vi "delete_curve.vi"(10 "簇":T23, 11 "配置":T1 {"串口通信UI"."Format" items=["标准帧", "扩展帧"]; "串口通信UI"."Type" items=["数据帧", "远程帧"]; "串口通信UI"."ID" format="0x%x"; "串口通信UI"."Fliter" items=["接收所有类型"=1, "只接收标准帧"=2, "只接收扩展帧"=3]; "串口通信UI"."kBaudRate" items=["5k bps"=1, "10k bps"=2, "20k bps"=3, "40k bps"=4, "50k bps"=5, "80k bps"=6, "100k bps"=7, "125k bps"=8, "200k bps"=9, "250k bps"=10, "400k bps"=11, "500k bps"=12, "666k bps"=13, "800k bps"=14, "1000k bps"=15, "33.33k bps"=16, "66.66k bps"=17, "83.33k bps"=18]; "串口通信UI"."Mode" items=["正常工作", "仅侦听模式", "自测模式（环回）"]; "串口通信UI"."InitFlag" items=["使用界面设置参数"=1]; "串口通信UI"."AccMask" format="%08x"; "串口通信UI"."AccCode" format="%08x"; "串口通信UI"."Channel" items=["通道1", "通道2"]; "串口通信UI"."DevType" items=["USB-CAN"=3, "USB-CAN2"=4]; "安全报警UI"."操作 8" items=["产生报警信息（不发声），等待手动操作", "产生报警信息（发声），等待手动操作", "产生报警信息（不发声），自动刹车", "产生报警信息（发声），自动刹车", "产生报警信息（不发声），立即自动断电，开启泄放电阻", "产生报警信息（发声），立即自动断电，开启泄放电阻"]; "安全报警UI"."操作 7" items=["产生报警信息（不发声），等待手动操作", "产生报警信息（发声），等待手动操作", "产生报警信息（不发声），自动刹车", "产生报警信息（发声），自动刹车", "产生报警信息（不发声），立即自动断电，开启泄放电阻", "产生报警信息（发声），立即自动断电，开启泄放电阻"]; "安全报警UI"."操作 6" items=["产生报警信息（不发声），等待手动操作", "产生报警信息（发声），等待手动操作", "产生报警信息（不发声），自动刹车", "产生报警信息（发声），自动刹车", "产生报警信息（不发声），立即自动断电，开启泄放电阻", "产生报警信息（发声），立即自动断电，开启泄放电阻"]; "安全报警UI"."操作 5" items=["产生报警信息（不发声），等待手动操作", "产生报警信息（发声），等待手动操作", "产生报警信息（不发声），自动刹车", "产生报警信息（发声），自动刹车", "产生报警信息（不发声），立即自动断电，开启泄放电阻", "产生报警信息（发声），立即自动断电，开启泄放电阻"]; "安全报警UI"."操作 4" items=["产生报警信息（不发声），等待手动操作", "产生报警信息（发声），等待手动操作", "产生报警信息（不发声），自动刹车", "产生报警信息（发声），自动刹车", "产生报警信息（不发声），立即自动断电，开启泄放电阻", "产生报警信息（发声），立即自动断电，开启泄放电阻"]; "安全报警UI"."操作 3" items=["产生报警信息（不发声），等待手动操作", "产生报警信息（发声），等待手动操作", "产生报警信息（不发声），自动刹车", "产生报警信息（发声），自动刹车", "产生报警信息（不发声），立即自动断电，开启泄放电阻", "产生报警信息（发声），立即自动断电，开启泄放电阻"]; "安全报警UI"."操作 2" items=["产生报警信息（不发声），等待手动操作", "产生报警信息（发声），等待手动操作", "产生报警信息（不发声），自动刹车", "产生报警信息（发声），自动刹车", "产生报警信息（不发声），立即自动断电，开启泄放电阻", "产生报警信息（发声），立即自动断电，开启泄放电阻"]; "安全报警UI"."操作" items=["产生报警信息（不发声），等待手动操作", "产生报警信息（发声），等待手动操作", "产生报警信息（不发声），自动刹车", "产生报警信息（发声），自动刹车", "产生报警信息（不发声），立即自动断电，开启泄放电阻", "产生报警信息（发声），立即自动断电，开启泄放电阻"]}) -> (3 "配置输出":T1 {"串口通信UI"."Format" items=["标准帧", "扩展帧"]; "串口通信UI"."Type" items=["数据帧", "远程帧"]; "串口通信UI"."ID" format="0x%x"; "串口通信UI"."Fliter" items=["接收所有类型"=1, "只接收标准帧"=2, "只接收扩展帧"=3]; "串口通信UI"."kBaudRate" items=["5k bps"=1, "10k bps"=2, "20k bps"=3, "40k bps"=4, "50k bps"=5, "80k bps"=6, "100k bps"=7, "125k bps"=8, "200k bps"=9, "250k bps"=10, "400k bps"=11, "500k bps"=12, "666k bps"=13, "800k bps"=14, "1000k bps"=15, "33.33k bps"=16, "66.66k bps"=17, "83.33k bps"=18]; "串口通信UI"."Mode" items=["正常工作", "仅侦听模式", "自测模式（环回）"]; "串口通信UI"."InitFlag" items=["使用界面设置参数"=1]; "串口通信UI"."AccMask" format="%08x"; "串口通信UI"."AccCode" format="%08x"; "串口通信UI"."Channel" items=["通道1", "通道2"]; "串口通信UI"."DevType" items=["USB-CAN"=3, "USB-CAN2"=4]; "安全报警UI"."操作 8" items=["产生报警信息（不发声），等待手动操作", "产生报警信息（发声），等待手动操作", "产生报警信息（不发声），自动刹车", "产生报警信息（发声），自动刹车", "产生报警信息（不发声），立即自动断电，开启泄放电阻", "产生报警信息（发声），立即自动断电，开启泄放电阻"]; "安全报警UI"."操作 7" items=["产生报警信息（不发声），等待手动操作", "产生报警信息（发声），等待手动操作", "产生报警信息（不发声），自动刹车", "产生报警信息（发声），自动刹车", "产生报警信息（不发声），立即自动断电，开启泄放电阻", "产生报警信息（发声），立即自动断电，开启泄放电阻"]; "安全报警UI"."操作 6" items=["产生报警信息（不发声），等待手动操作", "产生报警信息（发声），等待手动操作", "产生报警信息（不发声），自动刹车", "产生报警信息（发声），自动刹车", "产生报警信息（不发声），立即自动断电，开启泄放电阻", "产生报警信息（发声），立即自动断电，开启泄放电阻"]; "安全报警UI"."操作 5" items=["产生报警信息（不发声），等待手动操作", "产生报警信息（发声），等待手动操作", "产生报警信息（不发声），自动刹车", "产生报警信息（发声），自动刹车", "产生报警信息（不发声），立即自动断电，开启泄放电阻", "产生报警信息（发声），立即自动断电，开启泄放电阻"]; "安全报警UI"."操作 4" items=["产生报警信息（不发声），等待手动操作", "产生报警信息（发声），等待手动操作", "产生报警信息（不发声），自动刹车", "产生报警信息（发声），自动刹车", "产生报警信息（不发声），立即自动断电，开启泄放电阻", "产生报警信息（发声），立即自动断电，开启泄放电阻"]; "安全报警UI"."操作 3" items=["产生报警信息（不发声），等待手动操作", "产生报警信息（发声），等待手动操作", "产生报警信息（不发声），自动刹车", "产生报警信息（发声），自动刹车", "产生报警信息（不发声），立即自动断电，开启泄放电阻", "产生报警信息（发声），立即自动断电，开启泄放电阻"]; "安全报警UI"."操作 2" items=["产生报警信息（不发声），等待手动操作", "产生报警信息（发声），等待手动操作", "产生报警信息（不发声），自动刹车", "产生报警信息（发声），自动刹车", "产生报警信息（不发声），立即自动断电，开启泄放电阻", "产生报警信息（发声），立即自动断电，开启泄放电阻"]; "安全报警UI"."操作" items=["产生报警信息（不发声），等待手动操作", "产生报警信息（发声），等待手动操作", "产生报警信息（不发声），自动刹车", "产生报警信息（发声），自动刹车", "产生报警信息（不发声），立即自动断电，开启泄放电阻", "产生报警信息（发声），立即自动断电，开启泄放电阻"]})   [LabVIEW 2018, in "UI.lvlib"]
uses:
  UI.lvlib
  Settings/Settings.ctl
  Acquisition/Hardware Configuration.ctl
  Acquisition/Signal Type.ctl
  Logging/Logging Configuration.ctl
  Logging/Logging.lvlib
  Acquisition/Acquisition.lvlib
  Settings/Settings.lvlib
panel:
  # "参数配置文件"
  # "输入数据文件"
  # "加载电机"
  # "负载电机"
  # "注：每次运行实验时销毁现有所有图像"
  # "参数配置文件"
  # "输入数据文件"
  # "加载电机"
  # "负载电机"
  # "注：每次运行实验时销毁现有所有图像"
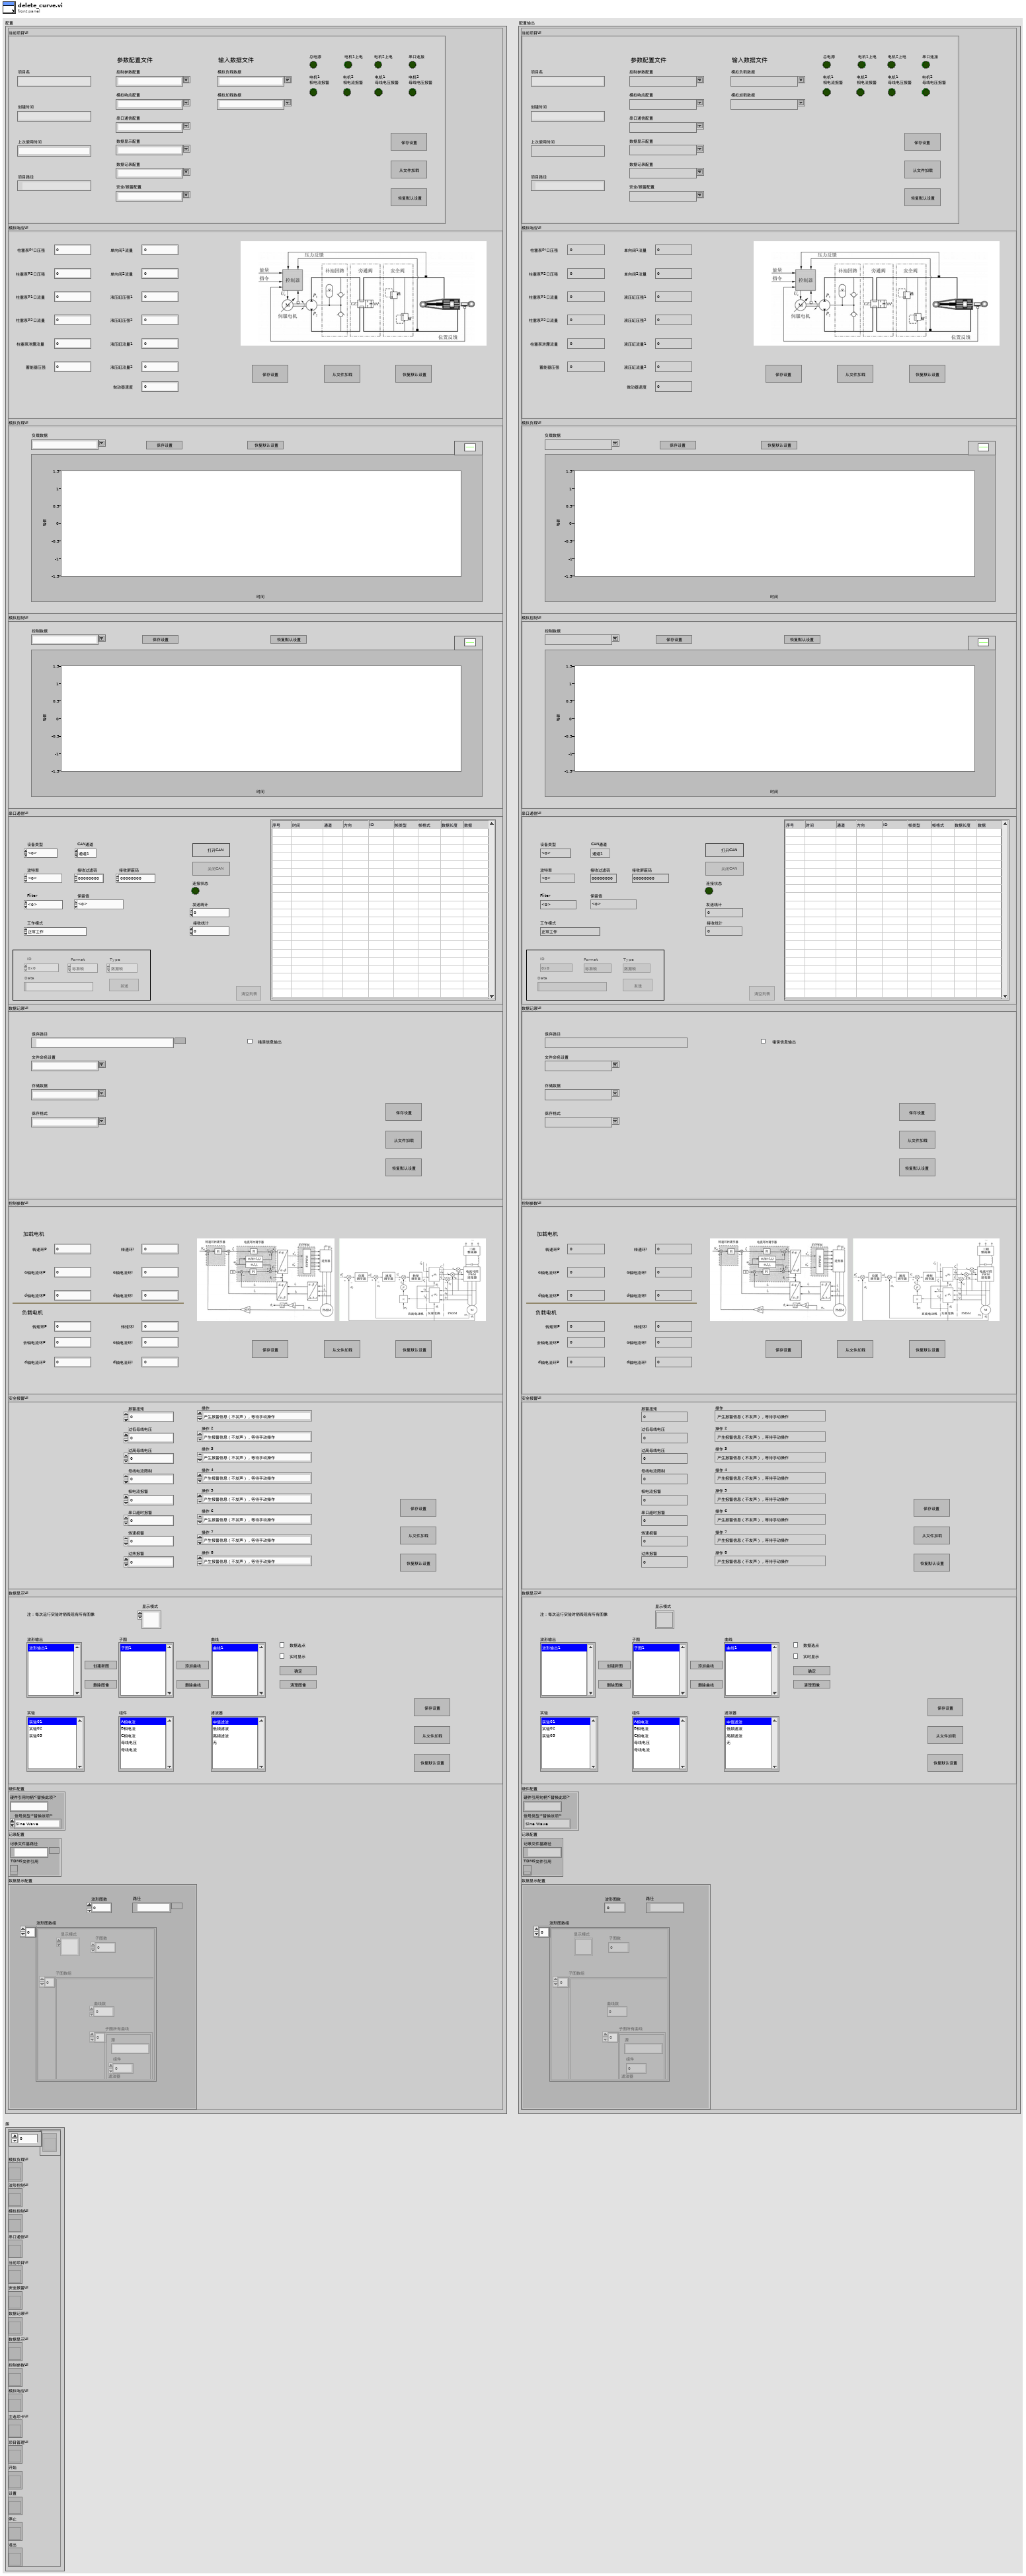
[diagram p1: front panel]
types:
  T1 = typedef "Settings.lvlib/Settings.ctl" = cluster{"当前项目UI":T2, "模拟响应UI":T3, "模拟负载UI":T4, "模拟控制UI":T5, "串口通信UI":T6, "数据记录UI":T12, "控制参数UI":T13, "安全报警UI":T14, "数据显示UI":T15, "硬件配置":T16, "记录配置":T18, "数据显示配置":T19}
  T2 = typedef "控件 5.ctl" = cluster{"控制参数配置":string, "模拟响应配置":string, "串口通信配置":string, "数据显示配置":string, "数据记录配置":string, "安全/报警配置":string, "模拟负载数据":string, "模拟加载数据":string, "总电源":bool, "电机1上电":bool, "电机2上电":bool, "串口连接":bool, "电机1\n相电流报警":bool, "电机2\n相电流报警":bool, "电机1\n母线电压报警":bool, "电机2\n母线电压报警":bool, "保存设置":bool, "从文件加载":bool, "恢复默认设置":bool, "路径":path, "项目路径":path, "项目名":string, "创建时间":string, "上次使用时间":string}
  T3 = typedef "模拟响应UI.ctl" = cluster{"柱塞泵P!口压强":dbl, "柱塞泵P2口压强":dbl, "柱塞泵P1口流量":dbl, "柱塞泵P2口流量":dbl, "柱塞泵泄露流量":dbl, "蓄能器压强":dbl, "单向阀1流量":dbl, "单向阀2流量":dbl, "液压缸压强1":dbl, "液压缸压强2":dbl, "液压缸流量1":dbl, "液压缸流量2":dbl, "做动器速度":dbl, "保存设置":bool, "从文件加载":bool, "恢复默认设置":bool, "路径":path}
  T4 = typedef "控件 9.ctl" = cluster{"负载数据":string, "负载数据 2":waveform(dbl)[], "保存设置":bool, "恢复默认设置":bool}
  T5 = typedef "控件 7.ctl" = cluster{"控制数据":string, "负载数据 2":waveform(dbl)[], "保存设置":bool, "恢复默认设置":bool}
  T6 = typedef "控件 6.ctl" = cluster{"DevType":T7, "Channel":T8, "AccCode":u32, "AccMask":u32, "InitFlag":T9, "Mode":T10, "kBaudRate":u8, "Fliter":T11, "Open":bool, "Close":bool, "连接状态":bool, "SendCnt":u32, "RecvCnt":u32, "Send":bool, "ID":u32, "Data":string, "Type":u8, "Format":u8, "Clear":bool, "list":i32, "路径":path}
  T7 = typedef "ControlCAN.lvlib/DevType.ctl" = u32
  T8 = typedef "ControlCAN.lvlib/CAN Channel.ctl" = u32
  T9 = typedef "ControlCAN.lvlib/InitFlag.ctl" = u32
  T10 = typedef "ControlCAN.lvlib/Mode.ctl" = u8
  T11 = typedef "ControlCAN.lvlib/Fliter.ctl" = u8
  T12 = typedef "控件 3.ctl" = cluster{"保存路径":path, "文件命名设置":string, "存储数据":string, "保存格式":string, "复选框":bool, "保存设置":bool, "从文件加载":bool, "恢复默认设置":bool, "路径":path}
  T13 = typedef "控件 1.ctl" = cluster{"d轴电流环P":dbl, "转速环P":dbl, "q轴电流环P":dbl, "d轴电流环P":dbl, "转矩环P":dbl, "去轴电流环P":dbl, "转速环I":dbl, "q轴电流环I":dbl, "d轴电流环I":dbl, "转矩环I":dbl, "q轴电流环I":dbl, "d轴电流环I":dbl, "保存设置":bool, "从文件加载":bool, "恢复默认设置":bool, "路径":path}
  T14 = typedef "控件 4.ctl" = cluster{"报警扭矩":dbl, "过低母线电压":dbl, "过高母线电压":dbl, "母线电流限制":dbl, "相电流报警":dbl, "串口超时报警":dbl, "转速报警":dbl, "过热报警":dbl, "操作":u16, "操作 2":u16, "操作 3":u16, "操作 4":u16, "操作 5":u16, "操作 6":u16, "操作 7":u16, "操作 8":u16, "保存设置":bool, "从文件加载":bool, "恢复默认设置":bool, "路径":path}
  T15 = typedef "控件 2.ctl" = cluster{"保存设置":bool, "从文件加载":bool, "恢复默认设置":bool, "实验":i32, "波形输出":i32, "组件":i32, "曲线":i32, "滤波器":i32, "删除曲线":bool, "清理图像":bool, "添加曲线":bool, "数据选点":bool, "确定按钮":bool, "实时显示":bool, "子图":i32, "显示模式":u16, "路径":path, "删除图像":bool, "创建新图":bool}
  T16 = typedef "Acquisition.lvlib/Hardware Configuration.ctl" = cluster{"硬件引用句柄<替换此项>":string, "信号类型<替换该项>":T17}
  T17 = typedef "Acquisition.lvlib/Signal Type.ctl" = enum16{"Sine Wave", "Square with Noise"}
  T18 = typedef "Logging.lvlib/Logging Configuration.ctl" = cluster{"记录文件基路径":path, "TDMS文件引用":refnum<k34>}
  T19 = typedef "波形图簇.ctl" = cluster{"波形图数":u32, "波形图数组":T20[], "路径":path}
  T20 = typedef "波形图.ctl" = cluster{"显示模式":u16, "子图数":u32, "子图数组":T21[]}
  T21 = typedef "子图.ctl" = cluster{"子图所有曲线":T22[], "曲线数":u32}
  T22 = typedef "曲线簇.ctl" = cluster{"源":string, "组件":u32, "滤波器":string}
  T23 = typedef "引用簇.ctl" = cluster{"数组":refnum<vi>[], "模拟负载UI":refnum<vi>, "波形控制UI":refnum<vi>, "模拟控制UI":refnum<vi>, "串口通信UI":refnum<vi>, "当前项目UI":refnum<vi>, "安全报警UI":refnum<vi>, "数据记录UI":refnum<vi>, "数据显示UI":refnum<vi>, "控制参数UI":refnum<vi>, "模拟响应UI":refnum<vi>, "主选项卡UI":refnum<vi>, "项目管理UI":refnum<vi>, "开始":refnum<vi>, "设置":refnum<vi>, "停止":refnum<vi>, "退出":refnum<vi>}
  T24 = enum8{"Enabled", "Disabled", "Disabled and Grayed Out"}
  T25 = typedef "组件常量.ctl" = string[]
  T26 = typedef "滤波器常量.ctl" = string[]
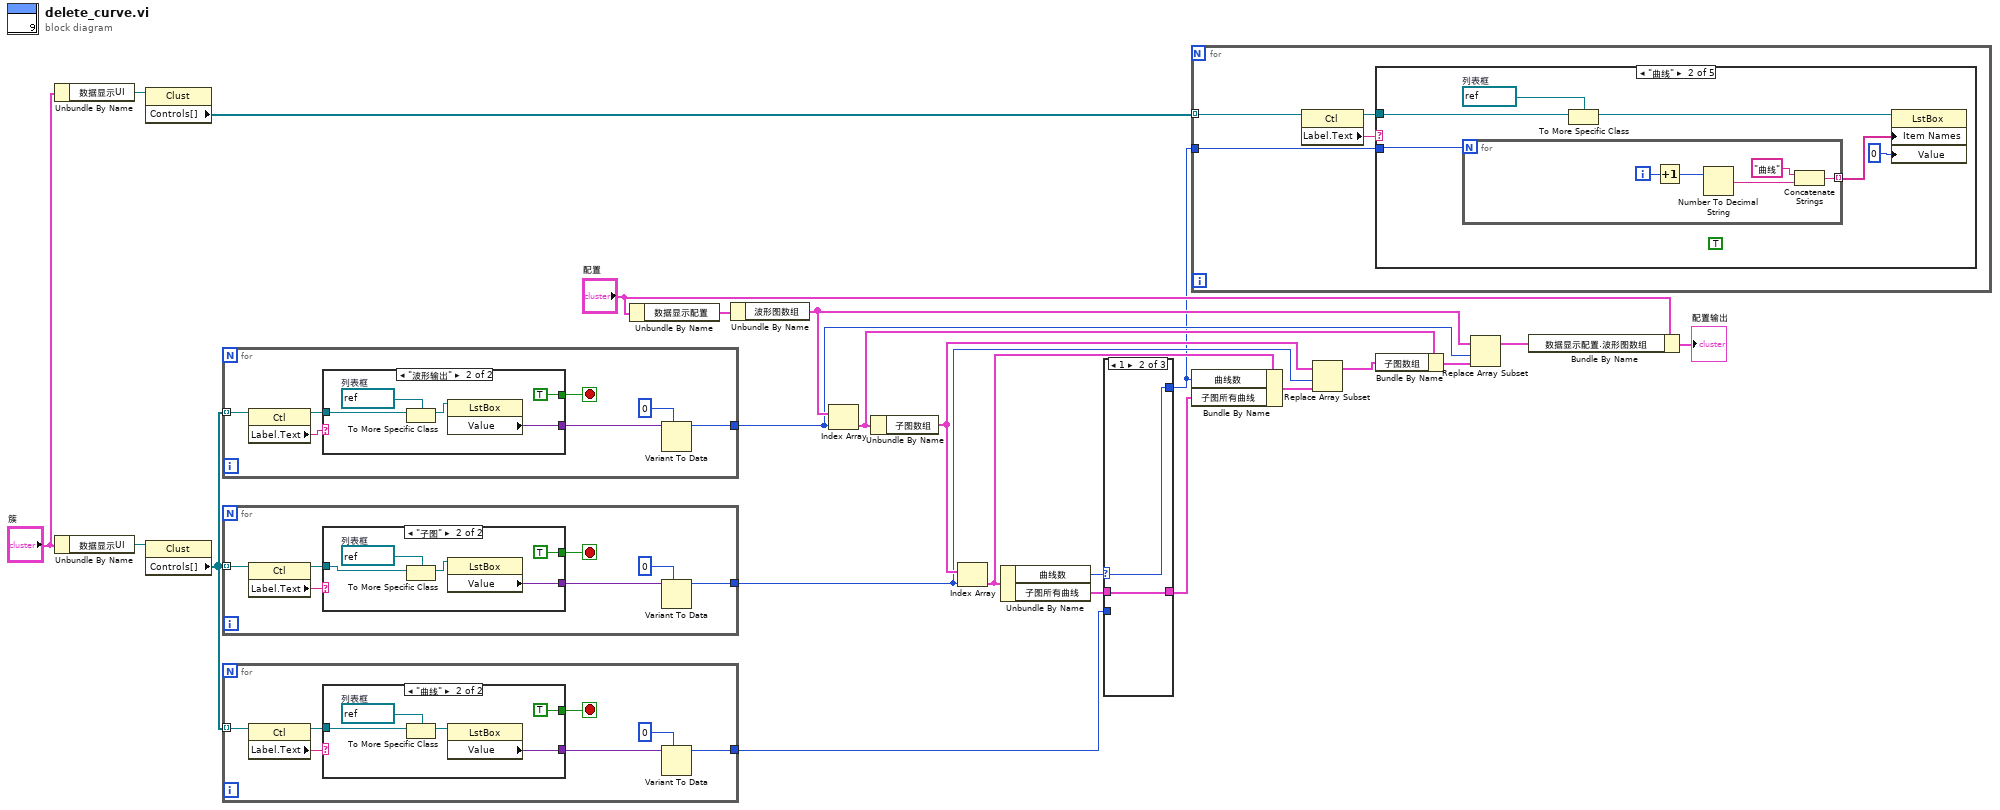
[diagram p0: block diagram]
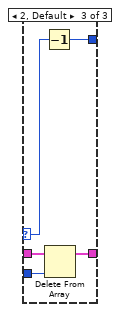
[diagram p3: hidden frame]
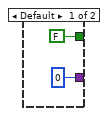
[diagram p4: hidden frame]
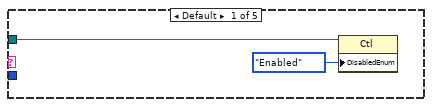
[diagram p5: hidden frame]
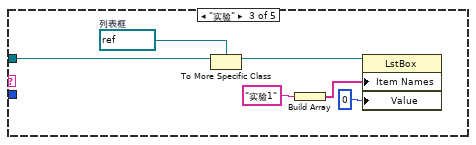
[diagram p6: hidden frame]
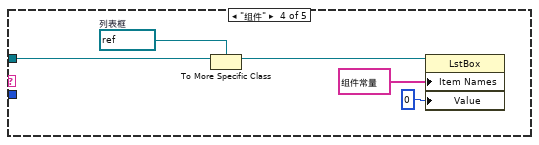
[diagram p7: hidden frame]
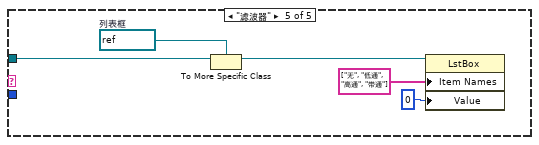
[diagram p8: hidden frame]
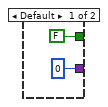
[diagram p9: hidden frame]
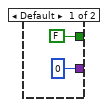
[diagram p10: hidden frame]
diagram:
  n1 = Unbundle By Name("簇") -> ("数据显示UI"=w10:refnum<vi>)
  n2 = Unbundle By Name("簇") -> ("数据显示UI"=w22:refnum<vi>)
  n3 = property class="Clust"(reference=w10) -> ("Controls[]"=w11:refnum<vi>[])  [unwired: 1 in, 2 out]
  n4 = property class="Clust"(reference=w22) -> ("Controls[]"=w6:refnum<vi>[])  [unwired: 1 in, 2 out]
  n5 = for {
    tunnel: [w27] -> w16
    tunnel: w6 -> [w24] mode=indexing
    stop <- w25 stop-if-true
    n6 = property class="Ctl"(reference=w24) -> (reference out=w29:refnum<vi>, "Label.Text"=w30:string)  [unwired: 1 in, 1 out]
    n7 = case shown="\"波形输出\"" w30 {
      tunnel: w29 -> [_ w37]
      tunnel: [0 w33] -> w28
      tunnel: [FALSE TRUE] -> w25
      frame Default {
      }
      frame "波形输出" {
        w36 = refnum<vi> refnum  # 列表框
        n8 = To More Specific Class(target class=w36, reference=w37) -> (specific class reference=w35:refnum<vi>)  [unwired: 1 in, 1 out]
        n9 = property class="LstBox"(reference=w35) -> ("Value"=w33:variant)  [unwired: 1 in, 2 out]
      }
    }
    n10 = Variant To Data(type=0, Variant=w28) -> (data=w27:i32)  [unwired: 1 in, 1 out]
  }
  n11 = for {
    tunnel: [w41] -> w20
    tunnel: w6 -> [w38] mode=indexing
    stop <- w39 stop-if-true
    n12 = property class="Ctl"(reference=w38) -> (reference out=w43:refnum<vi>, "Label.Text"=w44:string)  [unwired: 1 in, 1 out]
    n13 = case shown="\"子图\"" w44 {
      tunnel: w43 -> [_ w51]
      tunnel: [0 w47] -> w42
      tunnel: [FALSE TRUE] -> w39
      frame Default {
      }
      frame "子图" {
        w50 = refnum<vi> refnum  # 列表框
        n14 = To More Specific Class(target class=w50, reference=w51) -> (specific class reference=w49:refnum<vi>)  [unwired: 1 in, 1 out]
        n15 = property class="LstBox"(reference=w49) -> ("Value"=w47:variant)  [unwired: 1 in, 2 out]
      }
    }
    n16 = Variant To Data(type=0, Variant=w42) -> (data=w41:i32)  [unwired: 1 in, 1 out]
  }
  n17 = for {
    tunnel: [w55] -> w1
    tunnel: w6 -> [w52] mode=indexing
    stop <- w53 stop-if-true
    n18 = property class="Ctl"(reference=w52) -> (reference out=w57:refnum<vi>, "Label.Text"=w58:string)  [unwired: 1 in, 1 out]
    n19 = case shown="\"曲线\"" w58 {
      tunnel: w57 -> [_ w65]
      tunnel: [0 w61] -> w56
      tunnel: [FALSE TRUE] -> w53
      frame Default {
      }
      frame "曲线" {
        w64 = refnum<vi> refnum  # 列表框
        n20 = To More Specific Class(target class=w64, reference=w65) -> (specific class reference=w63:refnum<vi>)  [unwired: 1 in, 1 out]
        n21 = property class="LstBox"(reference=w63) -> ("Value"=w61:variant)  [unwired: 1 in, 2 out]
      }
    }
    n22 = Variant To Data(type=0, Variant=w56) -> (data=w55:i32)  [unwired: 1 in, 1 out]
  }
  n23 = Unbundle By Name("配置") -> ("数据显示配置"=w23:T19)
  n24 = Unbundle By Name(w23) -> ("波形图数组"=w17:T20[])
  n25 = Index Array(array=w17, index=w16) -> (element=w19:T20)
  n26 = Unbundle By Name(w19) -> ("子图数组"=w21:T21[])
  n27 = Index Array(array=w21, index=w20) -> (element=w8:T21)
  n28 = Unbundle By Name(w8) -> ("曲线数"=w2:u32, "子图所有曲线"=w5:T22[])
  n29 = case shown="1" w2 {
    selector: w2 -> [w66 w68 w70]
    tunnel: w5 -> [w67 w69 w74]
    tunnel: [w67 w69 w73] -> w4
    tunnel: [w66 w68 w72] -> w3
    tunnel: w1 -> [_ _ w71]
    frame 0 {
    }
    frame 1 {
    }
    frame 2, Default {
      n30 = Decrement(x=w70) -> (x-1=w72:u32)
      n31 = Delete From Array(array=w74, index=w71) -> (array with subset deleted=w73:T22[])  [unwired: 1 in, 1 out]
    }
  }
  n32 = for {
    tunnel: w11 -> [w78] mode=indexing
    tunnel: w3 -> [w75]
    n33 = property class="Ctl"(reference=w78) -> (reference out=w76:refnum<vi>, "Label.Text"=w77:string)  [unwired: 1 in, 1 out]
    n34 = case shown="\"曲线\"" w77 {
      tunnel: w76 -> [w80 w86 w97 w102 w107]
      tunnel: w75 -> [_ w83 _ _ _]
      frame Default {
        n35 = property class="Ctl"(reference=w80, "DisabledEnum"=T24."Enabled" ("禁用")) -> ()  [unwired: 1 in, 2 out]
      }
      frame "曲线" {
        (unwired) TRUE
        w85 = refnum<vi> refnum  # 列表框
        n36 = for {
          N: w83 -> [_]
          tunnel: [w87] -> w82 mode=indexing
          i -> [w91]
          n37 = Increment(x=w91) -> (x+1=w90:i32)
          n38 = Number To Decimal String(number=w90) -> (decimal integer string=w88:string)  [unwired: 1 in]
          n39 = Concatenate Strings("曲线", w88) -> (w87:string)
        }
        n40 = To More Specific Class(target class=w85, reference=w86) -> (specific class reference=w84:refnum<vi>)  [unwired: 1 in, 1 out]
        n41 = property class="LstBox"(reference=w84, "Item Names"=w82, "Value"=0) -> ()  [unwired: 1 in, 2 out]
      }
      frame "实验" {
        w96 = refnum<vi> refnum  # 列表框
        n42 = To More Specific Class(target class=w96, reference=w97) -> (specific class reference=w95:refnum<vi>)  [unwired: 1 in, 1 out]
        n43 = Build Array("实验1") -> (w94:string[])
        n44 = property class="LstBox"(reference=w95, "Item Names"=w94, "Value"=0) -> ()  [unwired: 1 in, 2 out]
      }
      frame "组件" {
        w101 = refnum<vi> refnum  # 列表框
        n45 = To More Specific Class(target class=w101, reference=w102) -> (specific class reference=w100:refnum<vi>)  [unwired: 1 in, 1 out]
        n46 = property class="LstBox"(reference=w100, "Item Names"=T25 ["正弦", "方波", "三角", "锯齿"] ("数组"), "Value"=0) -> ()  [unwired: 1 in, 2 out]
      }
      frame "滤波器" {
        w106 = refnum<vi> refnum  # 列表框
        n47 = To More Specific Class(target class=w106, reference=w107) -> (specific class reference=w105:refnum<vi>)  [unwired: 1 in, 1 out]
        n48 = property class="LstBox"(reference=w105, "Item Names"=T26 ["无", "低通", "高通", "带通"] ("数组"), "Value"=0) -> ()  [unwired: 1 in, 2 out]
      }
    }
  }
  n49 = Bundle By Name(cluster=w8, "曲线数"=w3, "子图所有曲线"=w4) -> (w7:T21)
  n50 = Replace Array Subset(array=w21, new element=w7, index=w20) -> (w18:T21[])
  n51 = Bundle By Name(cluster=w19, "子图数组"=w18) -> (w15:T20)
  n52 = Replace Array Subset(array=w17, new element=w15, index=w16) -> (w14:T20[])
  n53 = Bundle By Name(cluster="配置", "数据显示配置.波形图数组"=w14) -> (→"配置输出":T1)
